vi "Data Query.vi"(8 "error in (no error)":errorcluster, 11 "Modbus in":refnum<class "Modbus.lvclass">) -> (0 "error out":errorcluster, 3 "Modbus out":refnum<class "Modbus.lvclass">)   [LabVIEW 2020, in "Modbus.lvlib" / "Modbus.lvclass"]
uses:
  Modbus.lvclass
  C:/Program Files (x86)/National Instruments/LabVIEW 2020/vi.lib/ActorFramework/Actor/Actor.lvclass
  <vilib>/ActorFramework/Message Enqueuer/Message Priority.ctl
  <vilib>/ActorFramework/Actor/Actor.lvclass/Actor.ctl
  <vilib>/ActorFramework/Message Enqueuer/Message Enqueuer.lvclass/Message Enqueuer.ctl
  Modbus.lvclass/Modbus.ctl
  GUI Messages/Get Data from Modbus Msg/Get Data from Modbus Msg.lvclass/Get Data from Modbus Msg.ctl
  Modbus Messages/Write to Module Msg/Write to Module Msg.lvclass/Write to Module Msg.ctl
  eb6cec04-bcae-44df-be8b-1bc9d96078a7.vi
  <vilib>/ActorFramework/Message Enqueuer/Init from Existing Queue.vi
  <vilib>/ActorFramework/Message Enqueuer/Enqueue.vi
  GUI Messages/Get Data from Modbus Msg/Get Data from Modbus Msg.lvclass
  C:/Program Files (x86)/National Instruments/LabVIEW 2020/vi.lib/ActorFramework/Message/Message.lvclass
  Modbus Messages/Write to Module Msg/Write to Module Msg.lvclass
  <vilib>/NI Modbus.llb/MB Serial Master Query Read Holding Registers (poly).vi
  <vilib>/ActorFramework/Message Priority Queue/Priority Enqueue.vi
  Sensor/Sensor/Sensor.lvclass
  <vilib>/ActorFramework/Message Enqueuer/Message Enqueuer.lvclass
  <vilib>/ErrorRing/Error Ring.xnode
  <vilib>/ActorFramework/Actor/Actor.lvclass
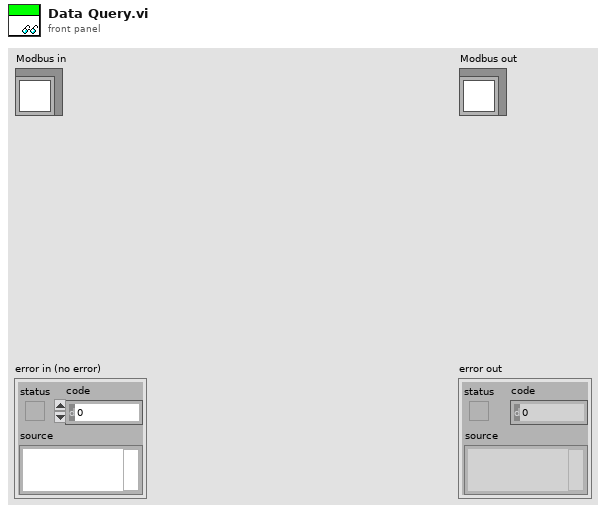
[diagram p1: front panel]
types:
  T1 = typedef "Actor Framework.lvlib/Message Enqueuer.lvclass/Message Priority.ctl" = enum16{"Low", "Normal", "High"}
  T2 = cluster{"Mode":enum16{"RTU", "ASCII"}, "Slave Address":u8}
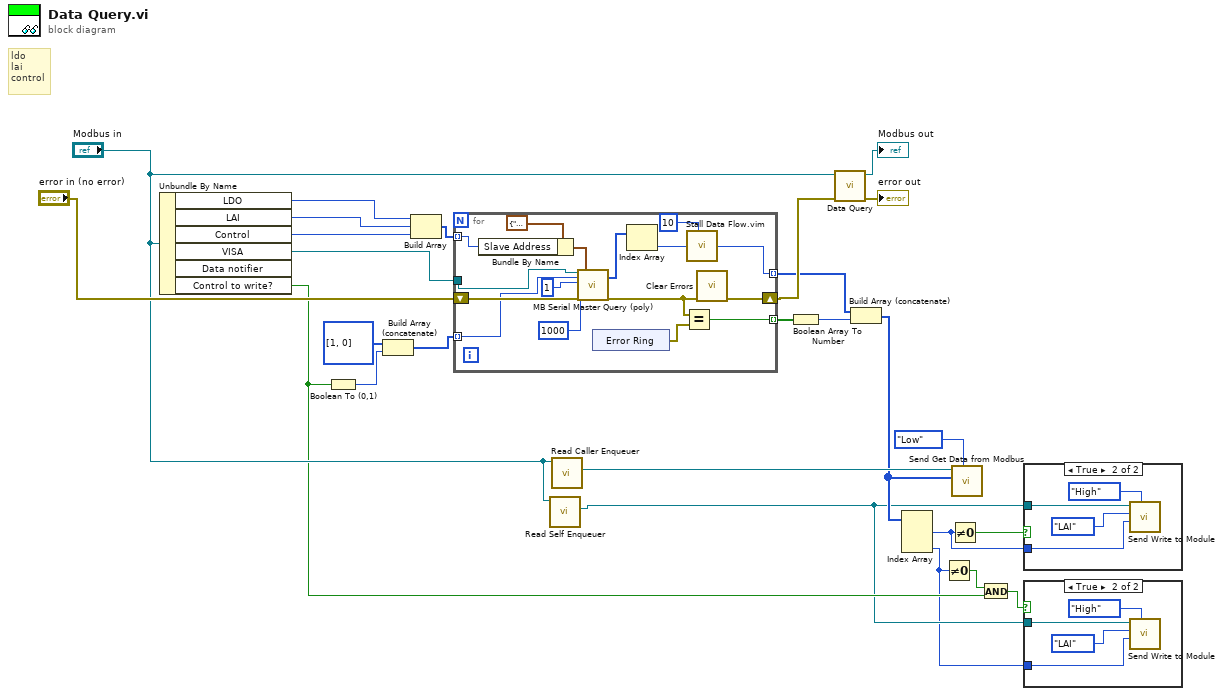
[diagram p0: block diagram]
diagram:
  # "ldo\nlai\ncontrol"
  n1 = Unbundle By Name("Modbus in") -> ("LDO"=w24:u16, "LAI"=w23:u16, "Control"=w13:u16, "VISA"=w18:refnum<visa-resource-name>, "Control to write?"=w4:bool)  [unwired: 1 out]
  n2 = Boolean To (0,1)(Boolean=w4) -> (0, 1=w12:i16)
  n3 = Build Array (concatenate)(u16[] [1, 0], w12) -> (w11:u16[])
  n4 = Build Array(w24, w23, w13) -> (w22:u16[])
  n5 = for {
    tunnel: w22 -> [w41] mode=indexing
    shift-right: [w34] -> w20
    shift-left: "error in (no error)" -> [w39]
    tunnel: [w29] -> w15 mode=indexing
    tunnel: w18 -> [w37]
    tunnel: [w35] -> w17 mode=indexing
    tunnel: w11 -> [w28] mode=indexing
    n6 = Bundle By Name(cluster=T2 {"Mode"=enum."RTU", "Slave Address"=0} ("Serial Parameters"), "Slave Address"=w41) -> (w40:T2)
    n7 = call-poly <vilib>:"MB Serial Master Query (poly).vi"("VISA resource name"=w37, "Starting Address"=w28, "Quantity"=u16 1 ("Starting Address"), "Timeout"=u32 1000, "error in"=w39, "Serial Parameters"=w40) -> ("Holding Registers"=w38:u16[], "error out"=w32:errorcluster)  [unwired: 10 in, 2 out]
    n8 = xnode "Error Ring"() -> ("error out"=w36:errorcluster)
    n9 = Index Array(array=w38) -> (element=w31:u16)  [unwired: 1 in]
    n10 = Equal?(x=w32, y=w36) -> (x = y?=w35:bool)
    n11 = call "Stall Data Flow.vim"("value in"=w31, "milliseconds to wait"=u32 10) -> ("value out"=w29:u16)  [unwired: 1 out]
    n12 = call <vilib>:"Clear Errors.vi"("error in (no error)"=w32) -> ("error out"=w34:errorcluster)  [unwired: 5 in, 1 out]
  }
  n13 = call <vilib>:"Read Self Enqueuer.vi"("Actor"="Modbus in") -> ("Self Enqueuer"=w2:refnum<class "Message Enqueuer.lvclass">)  [unwired: 10 in]
  n14 = call <vilib>:"Read Caller Enqueuer.vi"("Actor"="Modbus in") -> ("Caller Enqueuer"=w19:refnum<class "Message Enqueuer.lvclass">)  [unwired: 10 in]
  n15 = Boolean Array To Number(Boolean array=w17) -> (number=w16:u32)
  n16 = call-parent "Data Query.vi"("error in (no error)"=w20, "Sensor in"="Modbus in") -> ("error out"=→"error out":errorcluster, "Sensor out"=→"Modbus out":refnum<class "Modbus.lvclass">)  [unwired: 8 in]
  n17 = Build Array (concatenate)(w15, w16) -> (w9:u32[])
  n18 = Index Array(array=w9) -> (element #1=w6:u32, element #3=w1:u32)  [unwired: 3 in, 1 out]
  n19 = Not Equal To 0?(x=w1) -> (x != 0?=w5:bool)
  n20 = Not Equal To 0?(x=w6) -> (x != 0?=w8:bool)
  n21 = call "Send Get Data from Modbus.vi"("Message Priority (Normal)"=Message_Priority."Low", "Data"=w9, "Message Enqueuer"=w19) -> ()  [unwired: 7 in, 2 out]
  n22 = And(x=w5, y=w4) -> (x .and. y?=w3:bool)
  n23 = case shown="True" w8 {
    tunnel: w2 -> [_ w47]
    tunnel: w6 -> [_ w44]
    frame False {
    }
    frame True {
      n24 = call "Send Write to Module.vi"("Message Priority (Normal)"=Message_Priority."High", "Data"=w44, "Module"=enum16{"LAI", "LDO", "Control"}."LAI", "Message Enqueuer"=w47) -> ()  [unwired: 6 in, 2 out]
    }
  }
  n25 = case shown="True" w3 {
    tunnel: w1 -> [_ w49]
    tunnel: w2 -> [_ w48]
    frame False {
    }
    frame True {
      n26 = call "Send Write to Module.vi"("Message Priority (Normal)"=Message_Priority."High", "Data"=w49, "Module"=enum16{"LAI", "LDO", "Control"}."LAI", "Message Enqueuer"=w48) -> ()  [unwired: 6 in, 2 out]
    }
  }
